vi "0037-Sub_save.vi"(1 "部分配列 2":dbl[](array[numeric])) -> (7 "パス":path, 10 "転置配列":dbl[][](array[numeric]))   [LabVIEW 2014]
panel:
  out "部分配列":dbl[](array[numeric])
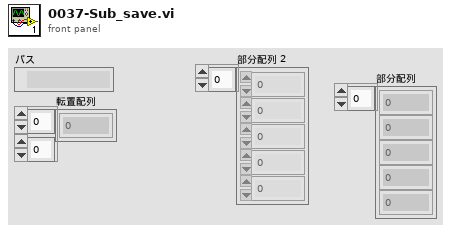
[diagram p1: front panel]
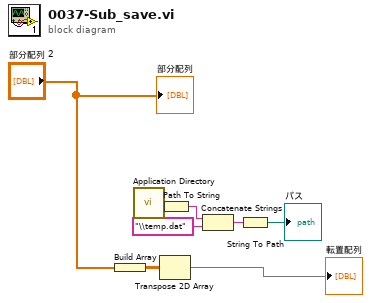
[diagram p0: block diagram]
diagram:
  n1 = Build Array("部分配列 2") -> (w4:dbl[][])
  n2 = call <vilib>:"Application Directory.vi"() -> ("Application Directory"=w6:path)
  n3 = Transpose 2D Array(2D array=w4) -> (transposed array=→"転置配列":dbl[][])
  n4 = Path To String(path=w6) -> (string=w7:string)
  n5 = Concatenate Strings(w7, "\\temp.dat" ("文字列")) -> (w8:string)
  n6 = String To Path(string=w8) -> (path=→"パス":path)
  "部分配列" <- "部分配列 2"
